vi "OpenFiles_Tree.vi"() -> ()   [LabVIEW 2018]
uses:
  HDF5/HDF5_ToneInfoClust.ctl
  <vilib>/addons/h5labview2/file/H5Fmode.ctl
  HDF5/HDF5_NoiseInfoClust.ctl
  HDF5/lib_path_mod_20200519.vi
  <vilib>/addons/h5labview2/base/H5Equery.vi
  <vilib>/addons/h5labview2/dataset/H5Dread.llb/H5Dread.xnode
  <vilib>/addons/h5labview2/file/H5F.lvlib
  <vilib>/addons/h5labview2/group/H5G.lvlib
  <vilib>/addons/h5labview2/dataset/H5D.lvlib
panel:
  out "data":T1[][](array[typedef])
  out "BrokenUpArray":string[][](array[string])
  out "names":string[][](array[string])
  out "Tree 2":string[](tree)
  in  "stop":bool
  in  "Tree":string[](tree)
  out "Folders":path[](array[path])
  out "Groups":string[](array[string])
  out "filenames":string[](array[string])
  in  "path":path
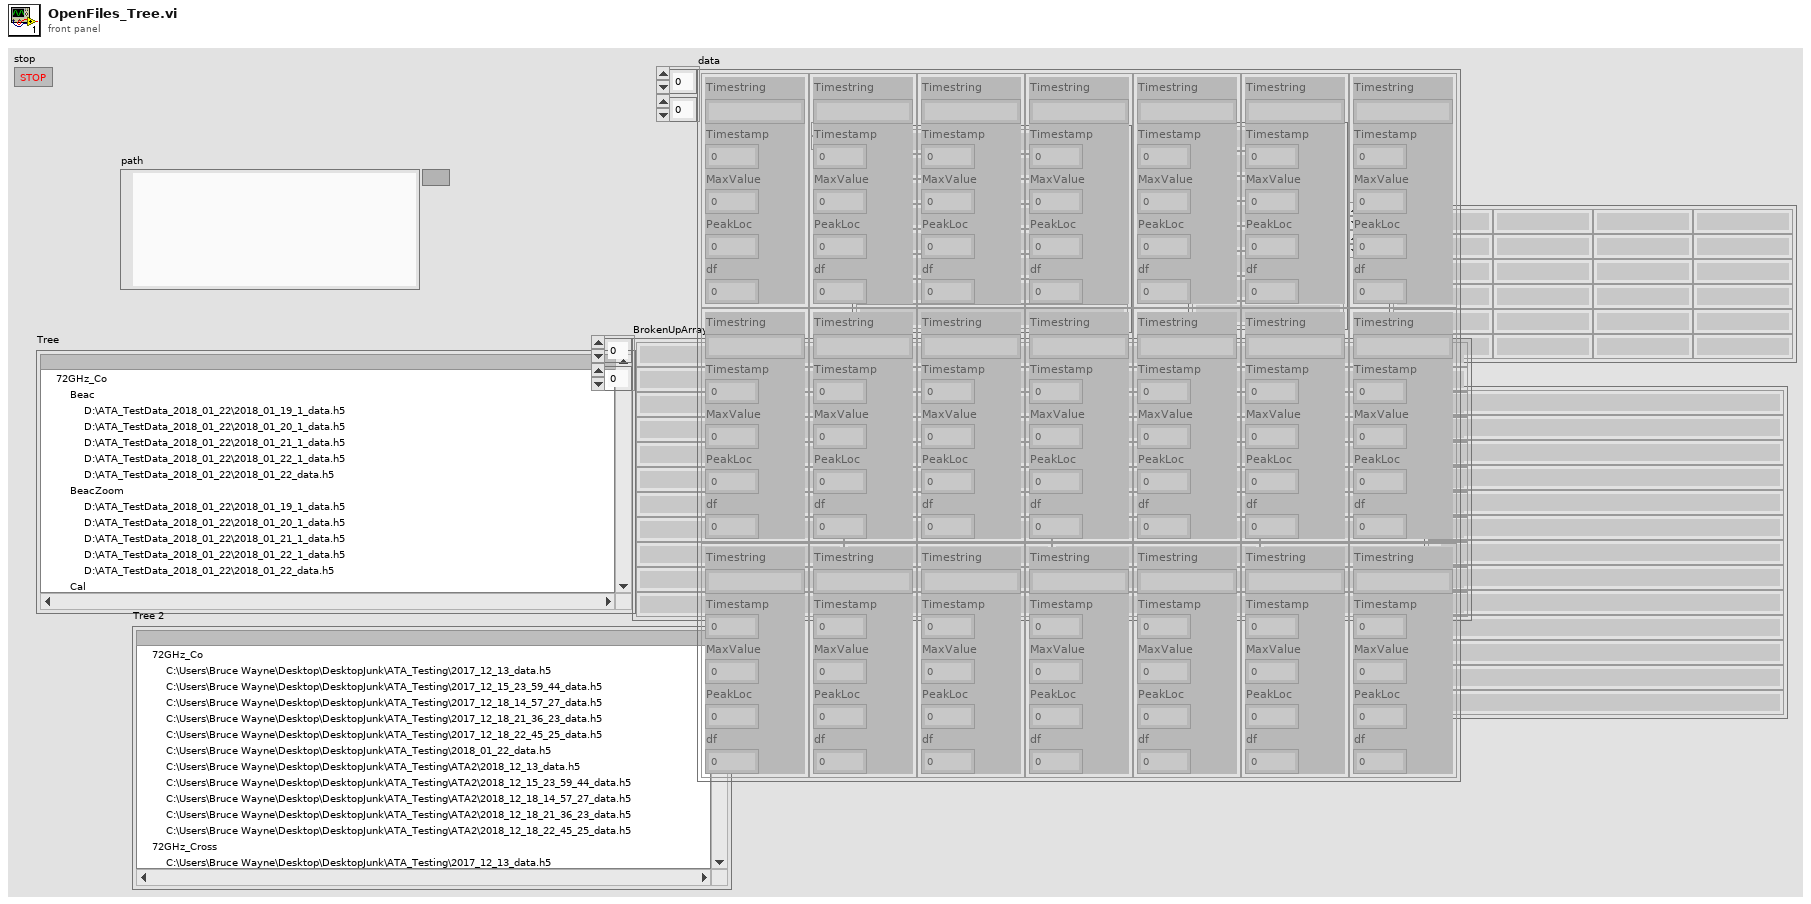
[diagram p1: front panel]
types:
  T1 = typedef "HDF5_ToneInfoClust.ctl" = cluster{"Timestring":string, "Timestamp":dbl, "MaxValue":dbl, "PeakLoc":dbl, "df":dbl}
  T2 = typedef "HDF5_NoiseInfoClust.ctl" = cluster{"Timestring":string, "Timestamp":dbl, "df":dbl, "Sum":dbl}
  T3 = typedef "H5F.lvlib/H5Fmode.ctl" = enum16{"read-only", "read-write", "overwrite", "create new", "open or create"}
  T4 = typedef "hid_t.ctl" = i32
  T5 = cluster{"Left Cell String":string, "Child Text":string[], "Child Tag":string, "Item Indent":i32, "Child Only?":bool, "Glyph Index":i32}
  T6 = cluster{"Left Cell String":string, "Child Text":string[], "Child Tag":string, "Item Indent":i32, "Child Only?":bool, "Glyph Index":i32}[]
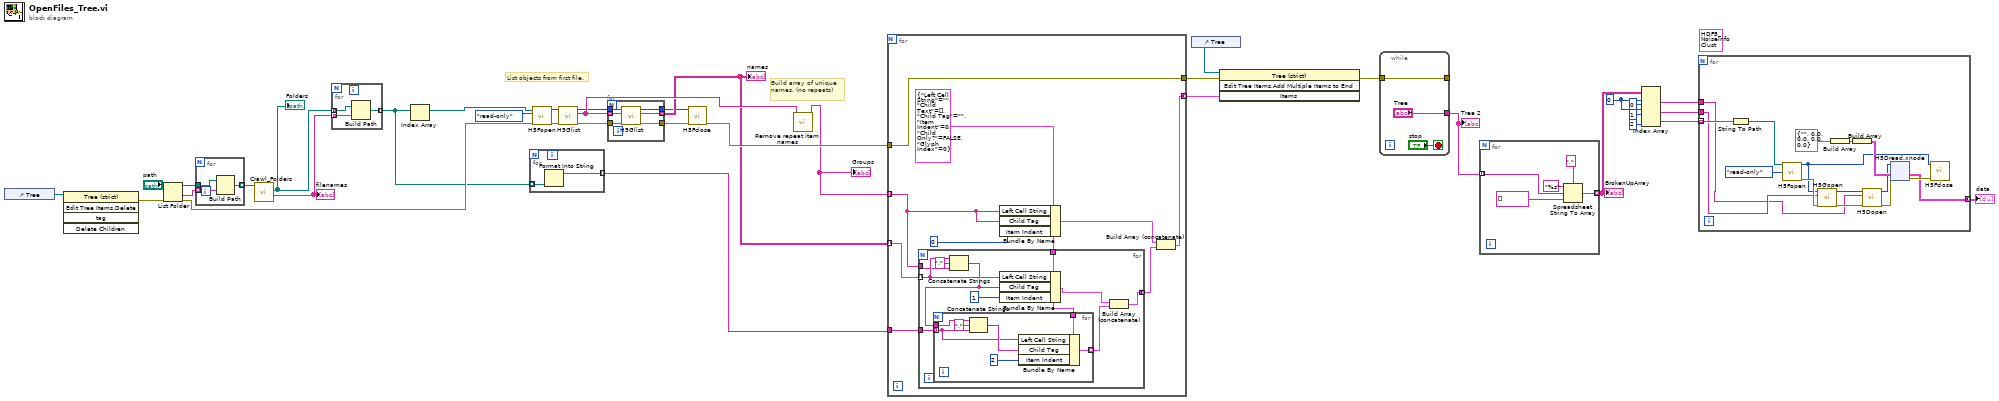
[diagram p0: block diagram]
diagram:
  w3 = 0 ("disabled index (row)")
  (unwired) T2 {"Timestring"="Timestamp string goes here", "Timestamp"=0.0, "df"=7629.39453125, "Sum"=0.0} ("HDF5_NoiseInfo")
  # "List objects from first file."
  # "Build array of unique names. (no repeats)"
  n1 = control-ref of="Tree"() -> (w29:refnum<vi>)
  n2 = invoke on="Invoke Node" class="Tree (strict)" method="Edit Tree Items.Delete"(reference=w29) -> (error out=w28:errorcluster)  [unwired: 4 in, 4 out]
  n3 = List Folder(path="path", error in=w28) -> (path out=w34:path, folder names=w35:string[], error out=w32:errorcluster)  [unwired: 2 in, 1 out]
  n4 = for {
    tunnel: w35 -> [w40] mode=indexing
    tunnel: w34 -> [w39]
    tunnel: [w38] -> w33 mode=indexing
    n5 = Build Path(base path=w39, name or relative path=w40) -> (appended path=w38:path)
  }
  n6 = call "Crawl_Folders.vi"("path in"=w33) -> ("FileNames"=w19:string[], "Folders"=w20:path[])  [unwired: 9 in]
  "filenames" <- w19
  "Folders" <- w20
  n7 = for {
    tunnel: w19 -> [w42] mode=indexing
    tunnel: w20 -> [w43] mode=indexing
    tunnel: [w41] -> w10 mode=indexing
    n8 = Build Path(base path=w43, name or relative path=w42) -> (appended path=w41:path)
  }
  n9 = Index Array(array=w10) -> (element=w11:path)  [unwired: 1 in]
  n10 = for {
    tunnel: w10 -> [w45] mode=indexing
    tunnel: [w44] -> w22 mode=indexing
    n11 = Format Into String(w45) -> (resulting string=w44:string)  [unwired: 3 in, 1 out]
  }
  n12 = call <vilib>:"H5Fopen.vi"("error in (no error)"=w32, "mode (read-only)"=H5Fmode."read-only" ("mode"), "path"=w11) -> ("error out"=w16:errorcluster, "ref out"=w17:T4)  [unwired: 7 in]
  n13 = call <vilib>:"H5Glist.vi"("error in (no error)"=w16, "ref in"=w17) -> ("error out"=w14:errorcluster, "names"=w37:string[], "ref out"=w15:T4)  [unwired: 6 in, 1 out]
  n14 = for {
    tunnel: w15 -> [w51]
    tunnel: w37 -> [w50] mode=indexing
    tunnel: w14 -> [w49]
    tunnel: [w48] -> w13
    tunnel: [w47] -> w12
    tunnel: [w46] -> w21 mode=indexing
    n15 = call <vilib>:"H5Glist.vi"("error in (no error)"=w49, "group (.)"=w50, "ref in"=w51) -> ("error out"=w48:errorcluster, "names"=w46:string[], "ref out"=w47:T4)  [unwired: 5 in, 1 out]
  }
  "names" <- w21
  n16 = call <vilib>:"H5Fclose.vi"("error in (no error)"=w13, "ref"=w12) -> ("error out"=w31:errorcluster)  [unwired: 9 in]
  n17 = call "Remove repeat item names.vi"("names"=w37) -> ("Array"=w30:string[])  [unwired: 10 in]
  "Groups" <- w30
  n18 = for {
    tunnel: w31 -> [w59]
    tunnel: w30 -> [w53] mode=indexing
    tunnel: w21 -> [w58] mode=indexing
    tunnel: [w55] -> w27 mode=concatenating
    tunnel: [w59] -> w25
    tunnel: w22 -> [w52]
    w54 = T5 {"Left Cell String"="", "Child Text"=[], "Child Tag"="", "Item Indent"=0, "Child Only?"=FALSE, "Glyph Index"=0} ("Item")
    n19 = for {
      tunnel: w58 -> [w69] mode=indexing
      tunnel: [w62] -> w57 mode=concatenating
      tunnel: w54 -> [w64]
      tunnel: w53 -> [w68]
      tunnel: w52 -> [w66]
      n20 = Concatenate Strings(w69, "," ("string"), w68) -> (w65:string)
      n21 = for {
        tunnel: w66 -> [w71] mode=indexing
        tunnel: w65 -> [w74]
        tunnel: w64 -> [w73]
        tunnel: [w72] -> w61 mode=indexing
        n22 = Concatenate Strings(w74, "," ("string"), w71) -> (w77:string)
        n23 = Bundle By Name(cluster=w73, "Left Cell String"=w71, "Child Tag"=w77, "Item Indent"=2) -> (w72:T5)
      }
      n24 = Bundle By Name(cluster=w64, "Left Cell String"=w69, "Child Tag"=w65, "Item Indent"=1) -> (w63:T5)
      n25 = Build Array (concatenate)(w63, w61) -> (w62:T6)
    }
    n26 = Bundle By Name(cluster=w54, "Left Cell String"=w53, "Child Tag"=w53, "Item Indent"=0) -> (w56:T5)
    n27 = Build Array (concatenate)(w56, w57) -> (w55:T6)
  }
  n28 = control-ref of="Tree"() -> (w26:refnum<vi>)
  n29 = invoke on="Invoke Node" class="Tree (strict)" method="Edit Tree Items.Add Multiple Items to End"(reference=w26, error in=w25, "Items"=w27) -> (error out=w24:errorcluster)  [unwired: 1 in, 3 out]
  n30 = while {
    tunnel: w24 -> [w80]
    tunnel: [w80] -> _
    tunnel: ["Tree"] -> w23
    stop <- "stop" stop-if-true
  }
  "Tree 2" <- w23
  n31 = for {
    tunnel: w23 -> [w85] mode=indexing
    tunnel: [w82] -> w9 mode=indexing
    n32 = Spreadsheet String To Array(delimiter (Tab)=",", format string="%s", spreadsheet string=w85, array type (2D Dbl)=string[] []) -> (array=w82:string[])
  }
  "BrokenUpArray" <- w9
  n33 = Index Array(array=w9, index (row) #1=w3, index (col) #1=0 ("disabled index (col)"), index (row) #2=w3, index (col) #2=1 ("index (col)"), index (col) #3=2 ("index (col)")) -> (element #1=w4:string, element #2=w2:string, element #3=w5:string[])  [unwired: 1 in]
  n34 = for {
    tunnel: w5 -> [w97] mode=indexing
    tunnel: w4 -> [w87]
    tunnel: w2 -> [w88]
    tunnel: [w89] -> w1 mode=concatenating
    n35 = String To Path(string=w97) -> (path=w96:path)
    n36 = call <vilib>:"H5Fopen.vi"("mode (read-only)"=H5Fmode."read-only" ("mode"), "path"=w96) -> ("error out"=w91:errorcluster, "ref out"=w86:T4)  [unwired: 8 in]
    n37 = call <vilib>:"H5Gopen.vi"("error in (no error)"=w91, "name"=w88, "ref in"=w86) -> ("error out"=w92:errorcluster, "group out"=w94:T4)  [unwired: 7 in]
    n38 = Build Array(T1 {"Timestring"="", "Timestamp"=0.0, "MaxValue"=0.0, "PeakLoc"=0.0, "df"=0.0} ("HDF5_ToneInfo in")) -> (w100:T1[])
    n39 = Build Array(w100) -> (w99:T1[][])
    n40 = call <vilib>:"H5Dopen.vi"("error in (no error)"=w92, "name"=w87, "loc in"=w94) -> ("error out"=w90:errorcluster, "dset out"=w93:T4)  [unwired: 7 in]
    n41 = xnode "H5Dread.xnode"("error in (no error)"=w90, "default"=w99, "ref in"=w93) -> ("error out"=w98:errorcluster, "data"=w89:T1[][])  [unwired: 3 in, 2 out]
    n42 = call <vilib>:"H5Fclose.vi"("error in (no error)"=w98, "ref"=w86) -> ()  [unwired: 9 in, 1 out]
  }
  "data" <- w1
